vi "File Exists.vi"(8 "error in":errorcluster, 11 "File Path":path) -> (0 "error out":errorcluster, 2 "Exists":bool, 3 "File Path (dup)":path)   [LabVIEW 2019, in "Open Xml.lvlib"]
uses:
  Open Xml.lvlib
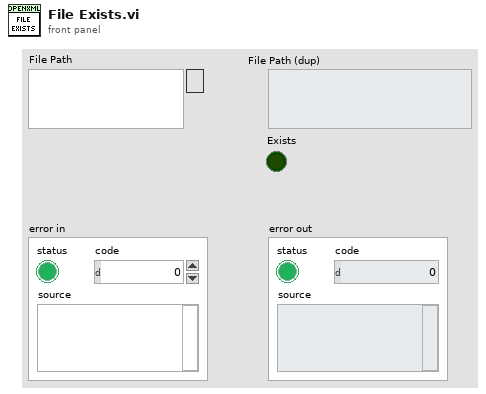
[diagram p1: front panel]
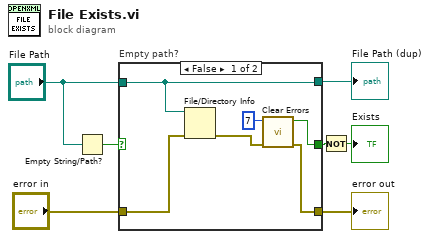
[diagram p0: block diagram]
diagram:
  n1 = Empty String/Path?(string/path="File Path") -> (empty?=w5:bool)
  n2 = case "Empty path?" shown="False" w5 {
    selector: w5 -> [_ w16]
    tunnel: "File Path" -> [w12 w15]
    tunnel: [w8 w14] -> w7
    tunnel: [w12 w15] -> w6
    tunnel: "error in" -> [w13 w14]
    tunnel: [w9 w16] -> w2
    frame False {
      n3 = File/Directory Info(path=w12, error in=w13) -> (error out=w11:errorcluster)  [unwired: 6 out]
      n4 = call <vilib>:"Clear Errors.vi"("error in (no error)"=w11, "specific error code to clear (0: all)"=7) -> ("error out"=w8:errorcluster, "specific error cleared?"=w9:bool)  [unwired: 4 in]
    }
    frame True {
    }
  }
  "error out" <- w7
  "File Path (dup)" <- w6
  n5 = Not(x=w2) -> (.not. x?=→"Exists":bool)
